vi "QMeter Select.vi"() -> (0 "Error":bool)   [LabVIEW 2010]
doc: "This VI writes to hardware to set the desired gain on a Yale card. The device, channel, and gain information is taken from the QCA Global."
uses:
  QCA Global.vi
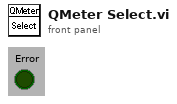
[diagram p1: front panel]
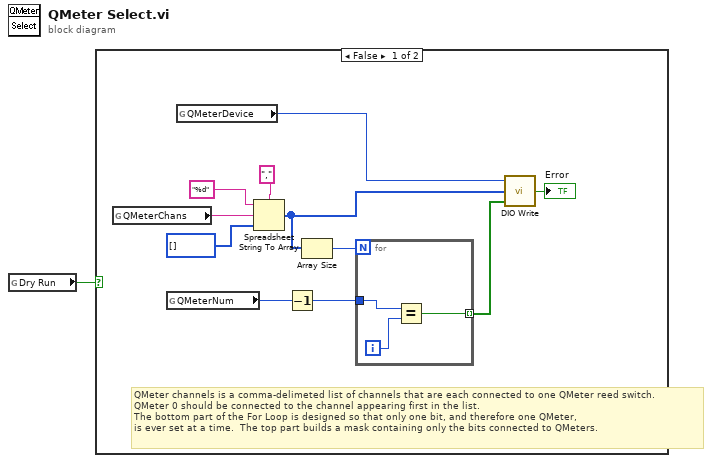
[diagram p0: block diagram]
diagram:
  n1 = global read "QCA Global.vi" "Dry Run"() -> (w1:bool)
  n2 = case shown="False" w1 {
    frame False {
      # "QMeter channels is a comma-delimeted list of channels that are each connected to one QMeter reed switch.\nQMeter 0 should be connected to the channel appearing first in the list.\nThe bottom part of the For Loop is designed so that only one bit, and therefore one QMeter,\nis ever set at a time.  The top part builds a mask containing only the bits connected to QMeters."
      n3 = global read "QCA Global.vi" "QMeterChans"() -> (w11:string)
      n4 = global read "QCA Global.vi" "QMeterNum"() -> (w5:i32)
      n5 = global read "QCA Global.vi" "QMeterDevice"() -> (w8:i32)
      n6 = Spreadsheet String To Array(delimiter (Tab)=",", format string="%d", spreadsheet string=w11, array type (2D Dbl)=i32[] [] ("Array Constant")) -> (array=w7:i32[])
      n7 = Decrement(x=w5) -> (x-1=w4:i32)
      n8 = Array Size(array=w7) -> (size(s)=w6:i32)
      n9 = for {
        N: w6 -> [_]
        tunnel: w4 -> [w15]
        tunnel: [w13] -> w3 mode=indexing
        i -> [w14]
        n10 = Equal?(x=w15, y=w14) -> (x = y?=w13:bool)
      }
      n11 = call "DIO Write.vi"("Data"=w3, "Channels"=w7, "device"=w8) -> ("Error"=→"Error":bool)
    }
    frame True {
    }
  }
